vi "Generate_FP_Snapshot.vi"(6 "TabControl in":refnum<vi>, 8 "error in":errorcluster, 11 "File_Name":path) -> (0 "error out":errorcluster)   [LabVIEW 2020]
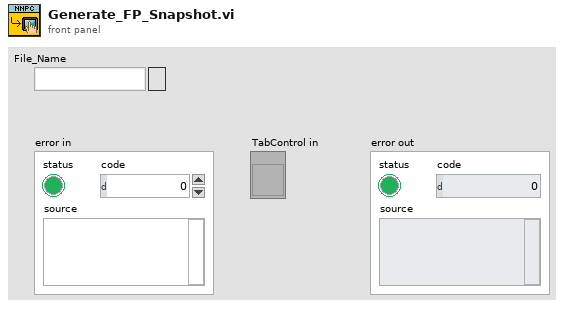
[diagram p1: front panel]
types:
  T1 = typedef "imagedata.ctl" = cluster{"image type":i32, "image depth":i32, "image":u8[], "mask":u8[], "colors":u32[], "Rectangle":cluster{"left":i16, "top":i16, "right":i16, "bottom":i16}}
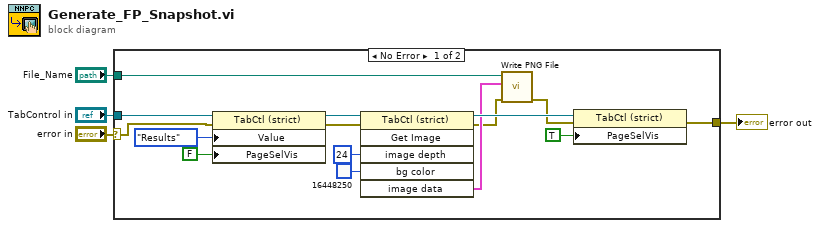
[diagram p0: block diagram]
diagram:
  n1 = case shown="No Error" "error in" {
    selector: "error in" -> [w18 w20]
    tunnel: "TabControl in" -> [w7 _]
    tunnel: "File_Name" -> [w5 _]
    tunnel: [w6 w20] -> w2
    frame No Error {
      n2 = property class="TabCtl (strict)"(reference=w7, error in=w18, "Value"=enum32{"Setup", "Results"}."Results", "PageSelVis"=FALSE ("Page Selector Visible")) -> (reference out=w12:refnum<vi>, error out=w13:errorcluster)
      n3 = invoke class="TabCtl (strict)" method="Get Image"(reference=w12, error in=w13, "image depth"=24 ("Image Depth"), "bg color"=u32 16448250 ("Background Color")) -> (reference out=w19:refnum<vi>, error out=w9:errorcluster, "image data"=w10:T1)  [unwired: 2 in, 3 out]
      n4 = call <vilib>:"Write PNG File.vi"("error in (no error)"=w9, "image data"=w10, "path to PNG file"=w5) -> ("error out"=w15:errorcluster)  [unwired: 7 in, 1 out]
      n5 = property class="TabCtl (strict)"(reference=w19, error in=w15, "PageSelVis"=TRUE ("Page Selector Visible")) -> (error out=w6:errorcluster)  [unwired: 1 out]
    }
    frame Error {
    }
  }
  "error out" <- w2
